vi "build_xwav.vi"(1 "x0 (0)":dbl, 2 "dx (1)":dbl=1.0, 3 "x units (index)":string="index", 4 "x dimention (x)":string="x", 7 "Y":dbl[](array[numeric]), 9 "y units (au)":string="au", 11 "attributes":variant) -> (8 "xwave":T1={"attributes"=variant, "X"={"start"=0.0, "delta"=0.0, "units"="index", "dim"="x"}, "Y"={"data"=[], "units"="au"}})   [LabVIEW 2015]
uses:
  xwav.ctl
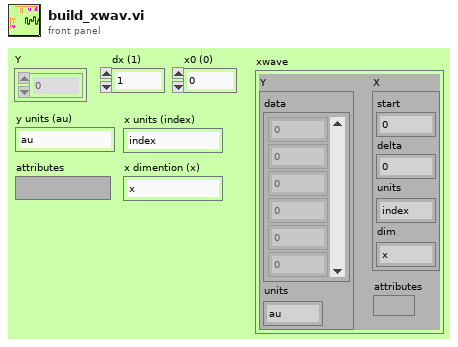
[diagram p1: front panel]
types:
  T1 = typedef "xwav.ctl" = cluster{"attributes":variant, "X":cluster{"start":dbl, "delta":dbl, "units":string, "dim":string}, "Y":cluster{"data":dbl[], "units":string}}
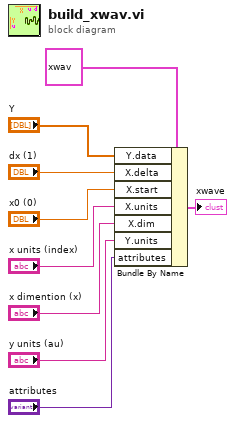
[diagram p0: block diagram]
diagram:
  n1 = Bundle By Name(cluster=T1 {"attributes"=variant, "X"={"start"=0.0, "delta"=0.0, "units"="index", "dim"="au"}, "Y"={"data"=[], "units"="au"}} ("xwave"), "Y.data"="Y", "X.delta"="dx (1)", "X.start"="x0 (0)", "X.units"="x units (index)", "X.dim"="x dimention (x)", "Y.units"="y units (au)", "attributes"="attributes") -> (→"xwave":T1)
